vi "Read DMD Calibration Parameter (SubVI).vi"() -> (3 "DMD Intensity Cal Param":T1)   [LabVIEW 2020]
uses:
  Controls (HOST)/DMD Intensity Cal Param.ctl
  <vilib>/Utility/config.llb/Read Key (Double).vi
  <vilib>/Utility/config.llb/Write Key (Double).vi
  <vilib>/Utility/config.llb/NI_LVConfig.lvlib
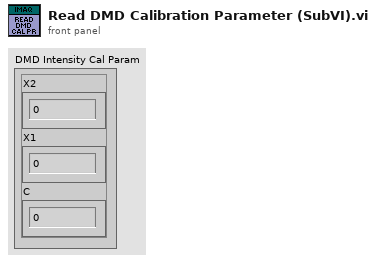
[diagram p1: front panel]
types:
  T1 = typedef "DMD Intensity Cal Param.ctl" = cluster{"X2":dbl, "X1":dbl, "C":dbl}
  T2 = typedef "NI_LVConfig.lvlib/Config Data RefNum.ctl" = refnum<k1>
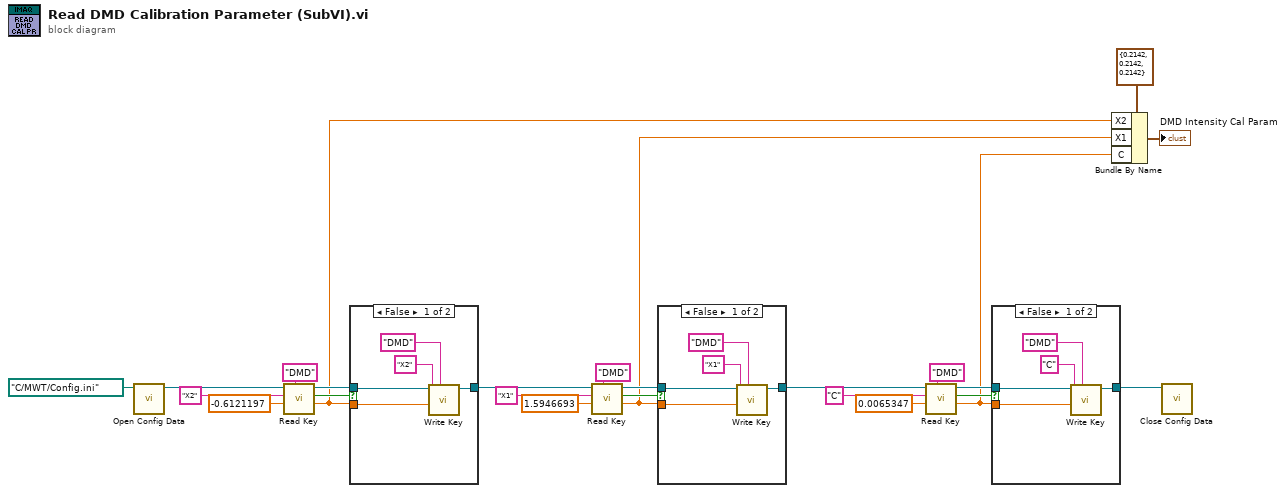
[diagram p0: block diagram]
diagram:
  n1 = call <vilib>:"Open Config Data.vi"("configuration file path"=path "C:/MWT/Config.ini") -> ("refnum"=w23:T2)  [unwired: 8 in, 2 out]
  n2 = call-poly <vilib>:"Read Key.vi"("section"="DMD", "default value"=-0.6121197, "key"="X2" ("section"), "refnum"=w23) -> ("value"=w3:dbl, "found?"=w22:bool, "refnum out"=w21:T2)  [unwired: 4 in, 1 out]
  n3 = case shown="False" w22 {
    tunnel: w21 -> [w28 w31]
    tunnel: [w27 w31] -> w14
    tunnel: w3 -> [w26 _]
    frame False {
      n4 = call-poly <vilib>:"Write Key.vi"("section"="DMD", "value"=w26, "key"="X2" ("section"), "refnum"=w28) -> ("refnum out"=w27:T2)  [unwired: 5 in, 2 out]
    }
    frame True {
    }
  }
  n5 = call-poly <vilib>:"Read Key.vi"("section"="DMD", "default value"=1.5946693, "key"="X1" ("section"), "refnum"=w14) -> ("value"=w4:dbl, "found?"=w17:bool, "refnum out"=w18:T2)  [unwired: 4 in, 1 out]
  n6 = case shown="False" w17 {
    tunnel: w18 -> [w34 w37]
    tunnel: [w33 w37] -> w7
    tunnel: w4 -> [w32 _]
    frame False {
      n7 = call-poly <vilib>:"Write Key.vi"("section"="DMD", "value"=w32, "key"="X1" ("section"), "refnum"=w34) -> ("refnum out"=w33:T2)  [unwired: 5 in, 2 out]
    }
    frame True {
    }
  }
  n8 = call-poly <vilib>:"Read Key.vi"("section"="DMD", "default value"=0.0065347, "key"="C" ("section"), "refnum"=w7) -> ("value"=w5:dbl, "found?"=w10:bool, "refnum out"=w11:T2)  [unwired: 4 in, 1 out]
  n9 = case shown="False" w10 {
    tunnel: w11 -> [w40 w43]
    tunnel: [w39 w43] -> w13
    tunnel: w5 -> [w38 _]
    frame False {
      n10 = call-poly <vilib>:"Write Key.vi"("section"="DMD", "value"=w38, "key"="C" ("section"), "refnum"=w40) -> ("refnum out"=w39:T2)  [unwired: 5 in, 2 out]
    }
    frame True {
    }
  }
  n11 = Bundle By Name(cluster=T1 {"X2"=0.2142, "X1"=0.2142, "C"=0.2142}, "X2"=w3, "X1"=w4, "C"=w5) -> (→"DMD Intensity Cal Param":T1)
  n12 = call <vilib>:"Close Config Data.vi"("refnum"=w13) -> ()  [unwired: 9 in, 2 out]
